vi "stimulate_and_record_async_time.vi"(3 "SSH password":string, 4 "Transfer and Run Date Folder After Experiment":bool, 5 "SSH user name":string, 6 "Tags":string, 7 "Frames":i32, 8 "Convert Power to Voltage":bool, 9 "voltages/power":dbl[](array[numeric]), 10 "parameters":string[](array[string]), 11 "parameters headers":string[](array[string])) -> ()   [LabVIEW 2016]
uses:
  <vilib>/vision/driver/IMAQdx.llb/IMAQdx Acquisition Mode.ctl
  <vilib>/userdefined/High Color/IMAQdx.ctl
  <vilib>/vision/driver/IMAQdx.llb/IMAQdx Buffer Number Mode.ctl
  <vilib>/Utility/file.llb/Write To Spreadsheet File (DBL).vi
  <vilib>/Utility/file.llb/Write To Spreadsheet File (string).vi
  <vilib>/Utility/file.llb/Read From Spreadsheet File (string).vi
  <vilib>/vision/driver/NI_Vision_Acquisition_Software.lvlib
panel:
  out "error out 2":errorcluster
  out "Saved Buffer Number":u32
  out "ProcessFrameRate":dbl
  out "# elements in queue":i32
  out "CameraFrameRate":dbl
  out "Camera Buffer Number":u32
  out "Image":T1(plugin-control)
  out "JPEG Quality":dbl
  out "Save Directory":path
  in  "stop":bool
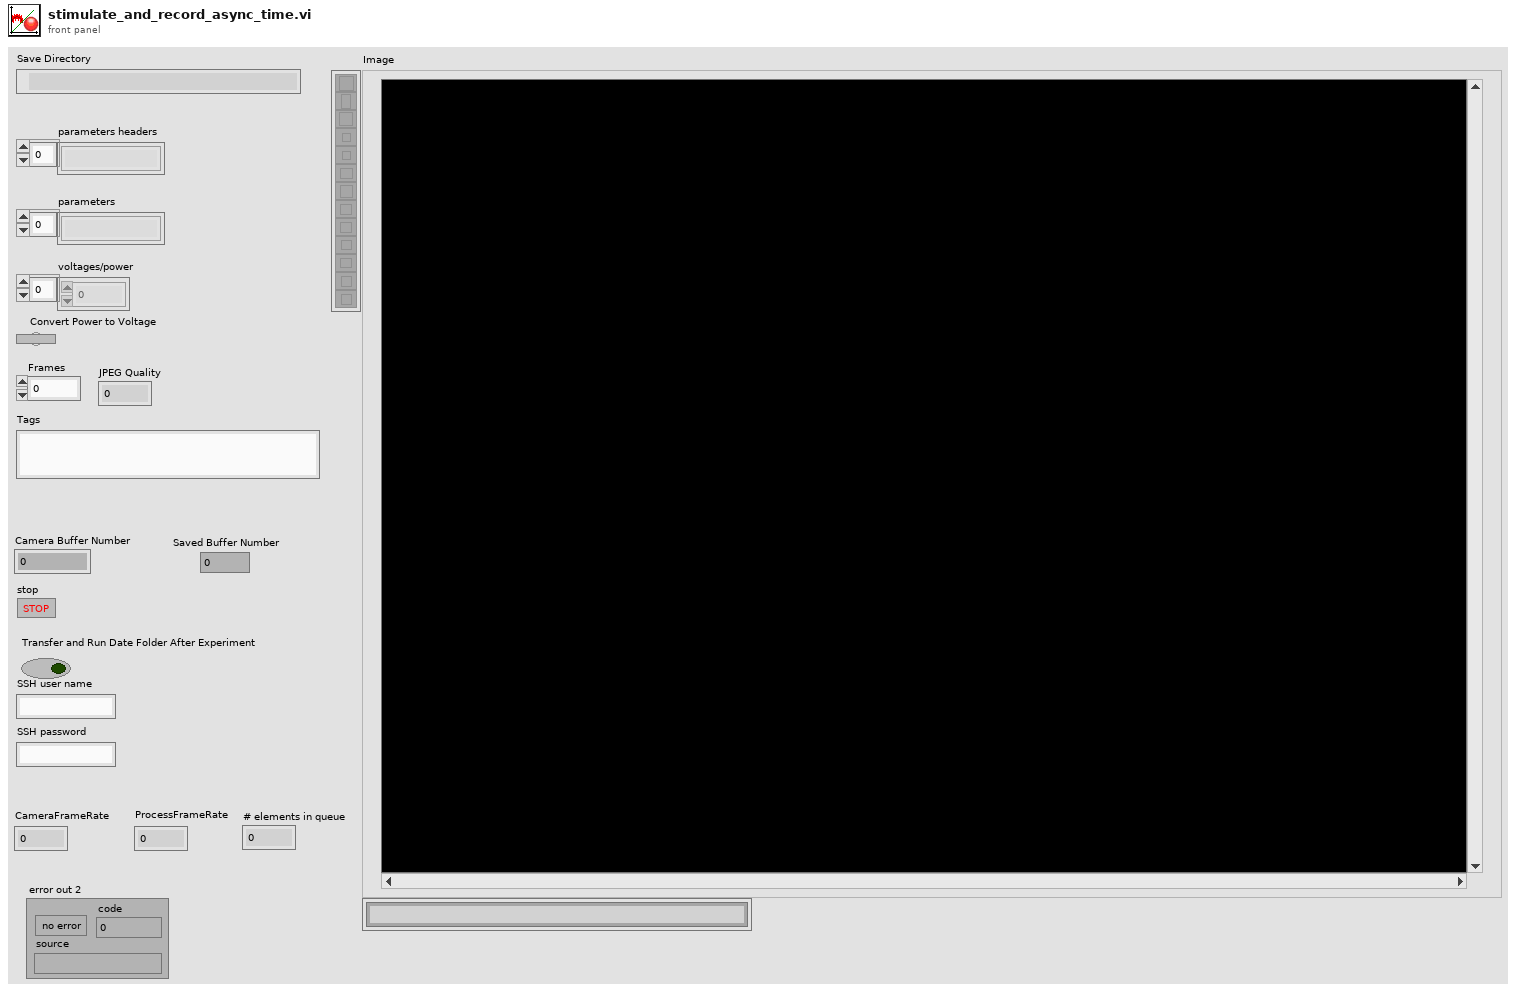
[diagram p1: front panel]
types:
  T1 = typedef "IMAQ Image.ctl" = refnum<image>
  T2 = typedef "IMAQdx.ctl" = refnum<k21>
  T3 = typedef "NI_Vision_Acquisition_Software.lvlib/IMAQdx Buffer Number Mode.ctl" = enum32{"Next", "Last", "Buffer Number", "Every", "Last New"}
  T4 = typedef "Image Type" = u32
  T5 = typedef "NI_Vision_Acquisition_Software.lvlib/IMAQdx Acquisition Mode.ctl" = enum32{"One Shot", "Continuous"}
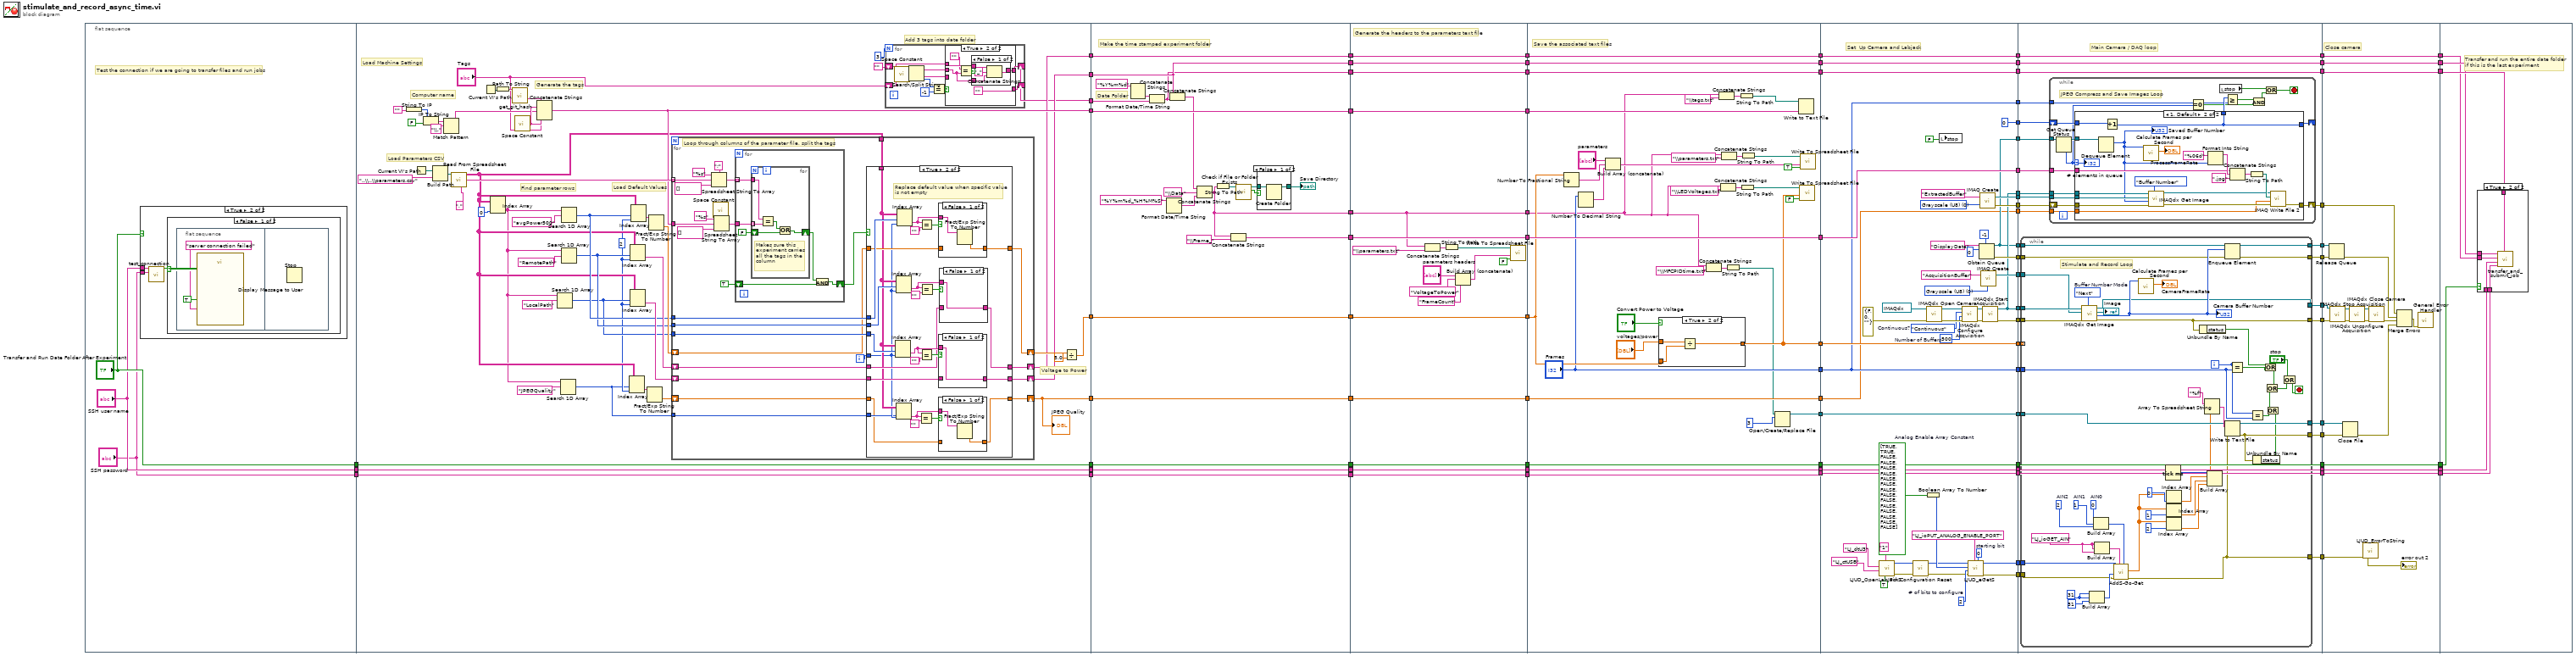
[diagram p0: block diagram]
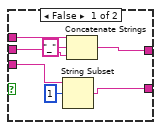
[diagram p4: hidden frame]
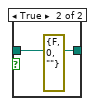
[diagram p11: hidden frame]
diagram:
  n1 = flat-sequence {
    tunnel: ["Transfer and Run Date Folder After Experiment"] -> w54
    tunnel: ["SSH user name"] -> w53
    tunnel: ["SSH password"] -> w52
    tunnel: [w136] -> w84
    tunnel: [w119] -> w83
    tunnel: [w110] -> w74
    tunnel: [w111] -> w73
    tunnel: w54 -> [w128]
    tunnel: w53 -> [w127]
    tunnel: w52 -> [w126]
    tunnel: [w128] -> w45
    tunnel: [w127] -> w38
    tunnel: [w126] -> w37
    tunnel: [w107] -> w30
    tunnel: [w98] -> w29
    tunnel: [w272] -> w68
    tunnel: [w271] -> w66
    tunnel: [w270] -> w64
    tunnel: [w269] -> w62
    tunnel: [w251] -> w60
    tunnel: [w253] -> w58
    tunnel: [w268] -> w56
    tunnel: w73 -> [w268]
    tunnel: w74 -> [w253]
    tunnel: w83 -> [w269]
    tunnel: w84 -> [w270]
    tunnel: [w260] -> w46
    tunnel: w45 -> [w260]
    tunnel: [w259] -> w39
    tunnel: w38 -> [w259]
    tunnel: w37 -> [w258]
    tunnel: [w258] -> w36
    tunnel: w30 -> [w254]
    tunnel: w29 -> [w250]
    tunnel: [w250] -> w26
    tunnel: w68 -> [w294]
    tunnel: [w294] -> w67
    tunnel: w66 -> [w280]
    tunnel: [w280] -> w65
    tunnel: w64 -> [w293]
    tunnel: [w293] -> w63
    tunnel: w62 -> [w292]
    tunnel: [w292] -> w61
    tunnel: w60 -> [w291]
    tunnel: [w291] -> w59
    tunnel: w58 -> [w290]
    tunnel: [w290] -> w57
    tunnel: w56 -> [w289]
    tunnel: [w289] -> w55
    tunnel: [w279] -> w47
    tunnel: w46 -> [w279]
    tunnel: [w278] -> w40
    tunnel: w39 -> [w278]
    tunnel: w36 -> [w277]
    tunnel: [w277] -> w35
    tunnel: [w276] -> w27
    tunnel: w26 -> [w276]
    tunnel: w67 -> [w327]
    tunnel: [w327] -> w89
    tunnel: [w311] -> w87
    tunnel: ["Frames"] -> w86
    tunnel: w65 -> [w295]
    tunnel: w63 -> [w307]
    tunnel: w61 -> [w302]
    tunnel: w59 -> [w316]
    tunnel: [w316] -> w79
    tunnel: [w315] -> w75
    tunnel: w57 -> [w315]
    tunnel: [w314] -> w69
    tunnel: w55 -> [w314]
    tunnel: [w305] -> w48
    tunnel: w47 -> [w305]
    tunnel: [w304] -> w41
    tunnel: w40 -> [w304]
    tunnel: w35 -> [w303]
    tunnel: [w303] -> w34
    tunnel: [w301] -> w28
    tunnel: w27 -> [w301]
    tunnel: [w299] -> w5
    tunnel: w89 -> [w356]
    tunnel: [w383] -> w88
    tunnel: w87 -> [w383]
    tunnel: w86 -> [w355]
    tunnel: [w355] -> w85
    tunnel: [w382] -> w80
    tunnel: w79 -> [w382]
    tunnel: [w381] -> w76
    tunnel: w75 -> [w381]
    tunnel: [w380] -> w70
    tunnel: w69 -> [w380]
    tunnel: [w379] -> w49
    tunnel: w48 -> [w379]
    tunnel: [w378] -> w42
    tunnel: w41 -> [w378]
    tunnel: w34 -> [w377]
    tunnel: [w377] -> w33
    tunnel: w28 -> [w353]
    tunnel: [w349] -> w25
    tunnel: [w357] -> w24
    tunnel: [w361] -> w23
    tunnel: [w360] -> w22
    tunnel: [w354] -> w21
    tunnel: [w359] -> w18
    tunnel: [w358] -> w17
    tunnel: [w357] -> w16
    tunnel: [w356] -> w15
    tunnel: [w355] -> w14
    tunnel: [w354] -> w13
    tunnel: [w353] -> w12
    tunnel: [0] -> w9
    tunnel: w5 -> [w350]
    tunnel: [w350] -> w4
    tunnel: [w339] -> w3
    tunnel: [w334] -> w1
    tunnel: w88 -> [w415]
    tunnel: w85 -> [w414]
    tunnel: [w413] -> w81
    tunnel: w80 -> [w413]
    tunnel: [w412] -> w77
    tunnel: w76 -> [w412]
    tunnel: [w411] -> w71
    tunnel: w70 -> [w411]
    tunnel: [w410] -> w50
    tunnel: w49 -> [w410]
    tunnel: [w409] -> w43
    tunnel: w42 -> [w409]
    tunnel: w33 -> [w408]
    tunnel: [w408] -> w32
    tunnel: w25 -> [w407]
    tunnel: w24 -> [w406]
    tunnel: w23 -> [w405]
    tunnel: w22 -> [w404]
    tunnel: w21 -> [w403]
    tunnel: [w402] -> w20
    tunnel: [w401] -> w19
    tunnel: w18 -> [w400]
    tunnel: w17 -> [w399]
    tunnel: w16 -> [w398]
    tunnel: w15 -> [w397]
    tunnel: w14 -> [w396]
    tunnel: w13 -> [w395]
    tunnel: w12 -> [w394]
    tunnel: [w391] -> w11
    tunnel: [w393] -> w10
    tunnel: w9 -> [w392]
    tunnel: [w390] -> w8
    tunnel: [w389] -> w7
    tunnel: [w388] -> w6
    tunnel: w4 -> [w387]
    tunnel: w3 -> [w386]
    tunnel: [w385] -> w2
    tunnel: w1 -> [w384]
    tunnel: [w526] -> w82
    tunnel: w81 -> [w526]
    tunnel: [w525] -> w78
    tunnel: w77 -> [w525]
    tunnel: [w524] -> w72
    tunnel: w71 -> [w524]
    tunnel: [w523] -> w51
    tunnel: w50 -> [w523]
    tunnel: [w522] -> w44
    tunnel: w43 -> [w522]
    tunnel: w32 -> [w521]
    tunnel: [w521] -> w31
    tunnel: w20 -> [w516]
    tunnel: w19 -> [w515]
    tunnel: w11 -> [w512]
    tunnel: w10 -> [w511]
    tunnel: w8 -> [w510]
    tunnel: w7 -> [w508]
    tunnel: w6 -> [w507]
    tunnel: w2 -> [w506]
    tunnel: w82 -> [w532]
    tunnel: w78 -> [w531]
    tunnel: w72 -> [w530]
    tunnel: w51 -> [w529]
    tunnel: w44 -> [w528]
    tunnel: w31 -> [w527]
    frame #0 {
      # "Test the connection if we are going to transfer files and run jobs"
      n2 = case shown="True" "Transfer and Run Date Folder After Experiment" {
        tunnel: "SSH password" -> [_ w95]
        tunnel: "SSH user name" -> [_ w93]
        frame False {
        }
        frame True {
          n3 = call "test_connection.vi"("Username"=w93, "Password"=w95) -> ("Connection Successful"=w94:bool)  [unwired: 7 in]
          n4 = case shown="False" w94 {
            frame False {
              n5 = flat-sequence {
                frame #0 {
                  n6 = call "Display Message to User"("Enable"=TRUE, "Message"="server connection failed") -> ()  [unwired: 8 in, 2 out]
                }
                frame #1 {
                  n7 = Stop() -> ()  [unwired: 1 in]
                }
              }
            }
            frame True {
            }
          }
        }
      }
    }
    frame #1 {
      w101 = 2
      # "Add 3 tags into date folder"
      # "Generate the tags"
      # "Find parameter rows"
      # "Load Default Values"
      # "Voltage to Power"
      # "Load Parameters CSV"
      # "Computer name"
      # "Load Machine Settings"
      n8 = String To IP(1:"") -> (0:w144:u32)
      n9 = Current VI's Path() -> (path=w139:path)
      n10 = IP To String(1:FALSE, 2:w144) -> (0:w141:string)
      n11 = Build Path(base path=w139, name or relative path="..\\..\\parameters.csv") -> (appended path=w130:path)
      n12 = Match Pattern(string=w141, regular expression="\\.") -> (before substring=w121:string)  [unwired: 1 in, 3 out]
      n13 = call-poly <vilib>:"Read From Spreadsheet File.vi"("delimiter (\\t)"=",", "file path (dialog if empty)"=w130) -> ("first row"=w120:string[], "all rows"=w103:string[][])  [unwired: 5 in, 3 out]
      n14 = Current VI's Path() -> (path=w123:path)
      n15 = Index Array(array=w103, index (col)=0) -> (element=w102:string[])  [unwired: 1 in]
      n16 = Path To String(path=w123) -> (string=w122:string)
      n17 = call "get_git_hash.vi"("VI folder"=w122) -> ("github hash"=w125:string)  [unwired: 10 in]
      n18 = call <vilib>:"Space Constant.vi"() -> ("String"=w124:string)
      n19 = Concatenate Strings(w125, w124, w121, w124, "Tags") -> (w119:string)
      n20 = Search 1D Array(1D array=w102, element="LocalPath") -> (index of element=w113:i32)  [unwired: 1 in]
      n21 = Search 1D Array(1D array=w102, element="JPEGQuality") -> (index of element=w99:i32)  [unwired: 1 in]
      n22 = Search 1D Array(1D array=w102, element="RemotePath") -> (index of element=w114:i32)  [unwired: 1 in]
      n23 = Search 1D Array(1D array=w102, element="avgPower500") -> (index of element=w115:i32)  [unwired: 1 in]
      n24 = Index Array(array=w103, index (row)=w99, index (col)=w101) -> (element=w104:string)
      n25 = Index Array(array=w103, index (row)=w114, index (col)=w101) -> (element=w117:string)
      n26 = Index Array(array=w103, index (row)=w113, index (col)=w101) -> (element=w116:string)
      n27 = Index Array(array=w103, index (row)=w115, index (col)=w101) -> (element=w132:string)
      n28 = Fract/Exp String To Number(string=w104) -> (number=w100:dbl)  [unwired: 3 in, 1 out]
      n29 = Fract/Exp String To Number(string=w132) -> (number=w118:dbl)  [unwired: 3 in, 1 out]
      n30 = for {
        tunnel: w120 -> [w198] mode=indexing
        tunnel: w119 -> [w190]
        tunnel: w115 -> [w185]
        tunnel: w114 -> [w184]
        tunnel: w113 -> [w183]
        tunnel: w103 -> [w188]
        shift-right: [w180] -> w112
        shift-left: w118 -> [w181]
        shift-right: [w177] -> w111
        shift-left: w117 -> [w178]
        shift-right: [w176] -> w110
        shift-left: w116 -> [w179]
        shift-right: [w173] -> w98
        shift-left: w100 -> [w175]
        tunnel: w99 -> [w174]
        i -> [w182]
        # "Loop through columns of the parameter file, split the tags"
        n31 = Spreadsheet String To Array(delimiter (Tab)=";", format string="%s", spreadsheet string=w198, array type (2D Dbl)=string[] []) -> (array=w194:string[])
        n32 = call <vilib>:"Space Constant.vi"() -> ("String"=w192:string)
        n33 = Spreadsheet String To Array(delimiter (Tab)=w192, format string="%s", spreadsheet string=w190, array type (2D Dbl)=string[] []) -> (array=w189:string[])
        n34 = for {
          tunnel: w194 -> [w244] mode=indexing
          tunnel: w189 -> [w243]
          shift-right: [w241] -> w186
          shift-left: TRUE -> [w239]
          n35 = for {
            tunnel: w244 -> [w249]
            tunnel: w243 -> [w248] mode=indexing
            shift-right: [w245] -> w240
            shift-left: FALSE -> [w246]
            # "Makes sure this\nexperiment carries\nall the tags in the\ncolumn"
            n36 = Equal?(x=w249, y=w248) -> (x = y?=w247:bool)
            n37 = Or(x=w247, y=w246) -> (x .or. y?=w245:bool)
          }
          n38 = And(x=w240, y=w239) -> (x .and. y?=w241:bool)
        }
        n39 = case shown="True" w186 {
          tunnel: w181 -> [w202 w223]
          tunnel: [w202 w222] -> w180
          tunnel: w185 -> [_ w228]
          tunnel: w184 -> [_ w227]
          tunnel: w183 -> [_ w226]
          tunnel: w182 -> [_ w205]
          tunnel: w188 -> [_ w206]
          tunnel: [w201 w212] -> w177
          tunnel: [w200 w214] -> w176
          tunnel: w179 -> [w200 w213]
          tunnel: w178 -> [w201 w211]
          tunnel: w175 -> [w199 w203]
          tunnel: w174 -> [_ w204]
          tunnel: [w199 w207] -> w173
          frame False {
          }
          frame True {
            # "Replace default value when specific value\nis not empty"
            n40 = Index Array(array=w206, index (row)=w226, index (col)=w205) -> (element=w215:string)
            n41 = Index Array(array=w206, index (row)=w227, index (col)=w205) -> (element=w218:string)
            n42 = Index Array(array=w206, index (row)=w204, index (col)=w205) -> (element=w208:string)
            n43 = Index Array(array=w206, index (row)=w228, index (col)=w205) -> (element=w221:string)
            n44 = Equal?(x=w208, y="") -> (x = y?=w209:bool)
            n45 = Equal?(x=w221, y="") -> (x = y?=w224:bool)
            n46 = Equal?(x=w215, y="") -> (x = y?=w216:bool)
            n47 = Equal?(x=w218, y="") -> (x = y?=w219:bool)
            n48 = case shown="False" w209 {
              tunnel: w203 -> [_ w231]
              tunnel: [w230 w231] -> w207
              tunnel: w208 -> [w229 _]
              frame False {
                n49 = Fract/Exp String To Number(string=w229) -> (number=w230:dbl)  [unwired: 3 in, 1 out]
              }
              frame True {
              }
            }
            n50 = case shown="False" w224 {
              tunnel: w223 -> [_ w238]
              tunnel: [w237 w238] -> w222
              tunnel: w221 -> [w236 _]
              frame False {
                n51 = Fract/Exp String To Number(string=w236) -> (number=w237:dbl)  [unwired: 3 in, 1 out]
              }
              frame True {
              }
            }
            n52 = case shown="False" w216 {
              tunnel: w215 -> [w232 _]
              tunnel: [w232 w233] -> w214
              tunnel: w213 -> [_ w233]
              frame False {
              }
              frame True {
              }
            }
            n53 = case shown="False" w219 {
              tunnel: w218 -> [w234 _]
              tunnel: [w234 w235] -> w212
              tunnel: w211 -> [_ w235]
              frame False {
              }
              frame True {
              }
            }
          }
        }
      }
      "JPEG Quality" <- w98
      n54 = for {
        N: 3 -> [_]
        shift-right: [w145] -> _
        shift-left: "Tags" -> [w154]
        shift-right: [w147] -> w107
        shift-left: "" -> [w152]
        n55 = call <vilib>:"Space Constant.vi"() -> ("String"=w153:string)
        n56 = Search/Split String(string=w154, search string/char (-)=w153) -> (substring before match=w151:string, match + rest of string=w150:string, offset of match=w149:i32)  [unwired: 1 in]
        n57 = Equal?(x=w149, y=-1) -> (x = y?=w146:bool)
        n58 = case shown="True" w146 {
          tunnel: w152 -> [w155 w165]
          tunnel: w151 -> [w156 w162]
          tunnel: w150 -> [w157 _]
          tunnel: [w159 ""] -> w145
          tunnel: [w158 w164] -> w147
          frame False {
            n59 = String Subset(string=w157, offset (0)=1) -> (substring=w159:string)  [unwired: 1 in]
            n60 = Concatenate Strings(w155, "_", w156) -> (w158:string)
          }
          frame True {
            n61 = Equal?(x="", y=w162) -> (x = y?=w166:bool)
            n62 = case shown="False" w166 {
              tunnel: w165 -> [w169 w172]
              tunnel: [w170 w172] -> w164
              tunnel: w162 -> [w168 _]
              frame False {
                n63 = Concatenate Strings(w169, "_", w168) -> (w170:string)
              }
              frame True {
              }
            }
          }
        }
      }
      n64 = Divide(x=w112, y=5.0) -> (x/y=w136:dbl)
    }
    frame #2 {
      # "Make the time stamped experiment folder"
      # "Date Folder"
      n65 = Format Date/Time String(time format string (%c)="%Y%m%d") -> (date/time string=w255:string)  [unwired: 2 in]
      n66 = Concatenate Strings(w255, w254) -> (w251:string)
      n67 = Format Date/Time String(time format string (%c)="%Y%m%d_%H%M%S") -> (date/time string=w257:string)  [unwired: 2 in]
      n68 = Concatenate Strings(w253, w251) -> (w252:string)
      n69 = Concatenate Strings(w252, "\\Data", w257) -> (w271:string)
      n70 = String To Path(string=w271) -> (path=w263:path)
      n71 = Concatenate Strings(w271, "\\Frame_") -> (w272:string)
      n72 = call <vilib>:"Check if File or Folder Exists.vi"("path"=w263) -> ("file or folder exists?"=w266:bool, "dup path"=w265:path)  [unwired: 8 in, 1 out]
      n73 = case shown="False" w266 {
        tunnel: [w273 w275] -> w262
        tunnel: w265 -> [w274 w275]
        frame False {
          n74 = Create Folder(path (use dialog)=w274) -> (created path=w273:path)  [unwired: 2 in, 2 out]
        }
        frame True {
          (unwired) errorcluster {"status"=FALSE, "code"=0, "source"=""} ("error out")
        }
      }
      "Save Directory" <- w262
    }
    frame #3 {
      # "Generate the headers to the parameters text file"
      n75 = Concatenate Strings(w280, "\\parameters.txt") -> (w288:string)
      n76 = String To Path(string=w288) -> (path=w287:path)
      n77 = Build Array (concatenate)("parameters headers", "VoltageToPower", "FrameCount") -> (w284:string[])
      n78 = call-poly <vilib>:"Write To Spreadsheet File.vi"("append to file? (new file:F)"=FALSE, "1D data"=w284, "file path (dialog if empty)"=w287) -> ()  [unwired: 5 in, 1 out]
    }
    frame #4 {
      # "Save the associated text files"
      n79 = Number To Fractional String(number=w307) -> (F-format string=w308:string)  [unwired: 3 in]
      n80 = Number To Decimal String(number="Frames") -> (decimal integer string=w309:string)  [unwired: 1 in]
      n81 = Build Array (concatenate)("parameters", w308, w309) -> (w320:string[])
      n82 = case shown="True" "Convert Power to Voltage" {
        tunnel: "voltages/power" -> [w330 w333]
        tunnel: [w330 w331] -> w311
        tunnel: w307 -> [_ w332]
        frame False {
        }
        frame True {
          n83 = Divide(x=w333, y=w332) -> (x/y=w331:dbl[])
        }
      }
      n84 = Concatenate Strings(w295, "\\MFCPIDtime.txt") -> (w298:string)
      n85 = Concatenate Strings(w295, "\\tags.txt") -> (w318:string)
      n86 = Concatenate Strings(w295, "\\LEDVoltages.txt") -> (w329:string)
      n87 = Concatenate Strings(w295, "\\parameters.txt") -> (w324:string)
      n88 = String To Path(string=w298) -> (path=w296:path)
      n89 = String To Path(string=w318) -> (path=w317:path)
      n90 = String To Path(string=w329) -> (path=w328:path)
      n91 = String To Path(string=w324) -> (path=w323:path)
      n92 = Open/Create/Replace File(file path (use dialog)=w296, operation (0:open)=3) -> (refnum out=w299:refnum<file>)  [unwired: 4 in, 2 out]
      n93 = Write to Text File(file (use dialog)=w317, text=w302) -> ()  [unwired: 2 in, 3 out]
      n94 = call-poly <vilib>:"Write To Spreadsheet File.vi"("append to file? (new file:F)"=FALSE, "1D data"=w311, "file path (dialog if empty)"=w328) -> ()  [unwired: 5 in, 1 out]
      n95 = call-poly <vilib>:"Write To Spreadsheet File.vi"("append to file? (new file:F)"=TRUE, "1D data"=w320, "file path (dialog if empty)"=w323) -> ()  [unwired: 5 in, 1 out]
    }
    frame #5 {
      w347 = 2  # # of bits to configure
      w345 = 0  # starting bit
      w344 = bool[] [TRUE, TRUE, FALSE, FALSE, FALSE, FALSE, FALSE, FALSE, FALSE, FALSE, FALSE, FALSE, FALSE, FALSE, FALSE, FALSE]  # Analog Enable Array Constant
      w364 = T4 0 items=["Grayscale (U8)", "Grayscale (I16)", "Grayscale (SGL)", "Complex (CSG)", "RGB (U32)", "HSL (U32)", "RGB (U64)"] ("Image Type")
      w373 = T4 0 items=["Grayscale (U8)", "Grayscale (I16)", "Grayscale (SGL)", "Complex (CSG)", "RGB (U32)", "HSL (U32)", "RGB (U64)"] ("Image Type")
      w374 = u32 500  # Number of Buffers
      w370 = IMAQdx_Acquisition_Mode."Continuous"  # Continuous?
      # "Set  Up Camera and Labjack"
      n96 = call "LJUD_OpenLabJackS.vi"("FirstFound"=TRUE, "Address"="1", "ConnectionType"="LJ_ctUSB", "DeviceType"="LJ_dtU3") -> ("error out"=w336:errorcluster, "Handle"=w338:i32)  [unwired: 5 in, 1 out]
      n97 = call "Pin Configuration Reset.vi"("error in"=w336, "Handle In"=w338) -> ("error out"=w335:errorcluster, "Handle Out"=w337:i32)  [unwired: 8 in]
      n98 = Boolean Array To Number(Boolean array=w344) -> (number=w348:u32)
      n99 = call <vilib>:"IMAQdx Open Camera.vi"("error in"=errorcluster {"status"=FALSE, "code"=0, "source"=""}, "Session In"=T2 "cam0") -> ("error out"=w375:errorcluster, "Session Out"=w376:T2)  [unwired: 8 in]
      n100 = local write "stop"(FALSE) -> ()
      n101 = call <vilib>:"IMAQdx Configure Acquisition.vi"("error in"=w375, "Number of Buffers"=w374, "Continuous?"=w370, "Session In"=w376) -> ("error out"=w371:errorcluster, "Session Out"=w369:T2)  [unwired: 6 in]
      n102 = call "LJUD_eGetS.vi"("Channel"=w345, "IOType"="LJ_ioPUT_ANALOG_ENABLE_PORT", "error in"=w335, "x1"=w347, "Value Write"=w348, "Handle In"=w337) -> ("error out"=w339:errorcluster, "Handle Out"=w334:i32)  [unwired: 3 in, 1 out]
      n103 = Obtain Queue(max queue size (-1, unlimited)=-1, name (unnamed)="DisplayData", element data type=u32 0) -> (queue out=w354:refnum<queue>, error out=w360:errorcluster)  [unwired: 2 in, 1 out]
      n104 = call "IMAQ Create"("Image Name"="ExtractedBuffer", "Image Type"=w364) -> ("New Image"=w358:T1, "error out"=w359:errorcluster)  [unwired: 3 in]
      n105 = call "IMAQ Create"("Image Name"="AcquisitionBuffer", "Image Type"=w373) -> ("New Image"=w361:T1)  [unwired: 3 in, 1 out]
      n106 = call <vilib>:"IMAQdx Start Acquisition.vi"("error in"=w371, "Session In"=w369) -> ("error out"=w349:errorcluster, "Session Out"=w357:T2)  [unwired: 8 in]
    }
    frame #6 {
      # "Main Camera / DAQ loop"
      n107 = while {
        tunnel: w415 -> [_] mode=indexing
        tunnel: w414 -> [w460]
        tunnel: w407 -> [w501]
        tunnel: w406 -> [w500]
        tunnel: w405 -> [w499]
        tunnel: w404 -> [w498]
        tunnel: w403 -> [w497]
        tunnel: [w494] -> w390
        tunnel: [w493] -> w391
        tunnel: [w492] -> w402
        tunnel: [w491] -> w401
        tunnel: [w465] -> w389
        tunnel: [w487] -> w388
        tunnel: w387 -> [w486]
        tunnel: w386 -> [w467]
        tunnel: [w466] -> w385
        tunnel: w384 -> [w456]
        i -> [w461]
        stop <- w459 stop-if-true
        w477 = 2  # AIN2
        w473 = 31 ("AIN0")
        w481 = 1  # AIN1
        w480 = 0  # AIN0
        w474 = "LJ_ioGET_AIN" ("IOType")
        w505 = IMAQdx_Buffer_Number_Mode."Next"  # Buffer Number Mode
        # "Stimulate and Record Loop"
        n108 = call <vilib>:"IMAQdx Get Image.vi"("Buffer Number Mode (Next)"=w505, "error in"=w501, "Image In"=w499, "Session In"=w500) -> ("error out"=w491:errorcluster, "Buffer Number Out"=w502:u32, "Image Out"=→"Image":T1, "Session Out"=w492:T2)  [unwired: 4 in]
        "Camera Buffer Number" <- w502
        n109 = Build Array(w473, w473, 31 ("AIN1")) -> (w478:i32[])
        n110 = Build Array(w480, w481, w477) -> (w484:i32[])
        n111 = Build Array(w474, w474, w474) -> (w485:string[])
        n112 = call "AddS-Go-Get.vi"("Channels"=w484, "IOTypes"=w485, "error in"=w467, "x1"=w478, "Handle In"=w456) -> ("error out"=w466:errorcluster, "Values Read"=w475:dbl[])  [unwired: 4 in, 1 out]
        n113 = call <vilib>:"Calculate Frames per Second.vi"("Buffer Number"=w502) -> ("Processed Frames/s"=→"CameraFrameRate":dbl)  [unwired: 8 in, 2 out]
        n114 = Tick Count (ms)() -> (millisecond timer value=w472:u32)
        n115 = Index Array(array=w475, index=0 ("Index")) -> (element=w470:dbl)
        n116 = Index Array(array=w475, index=1 ("Index")) -> (element=w469:dbl)
        n117 = Index Array(array=w475, index=2 ("Index")) -> (element=w468:dbl)
        n118 = Unbundle By Name(w491) -> ("status"=w496:bool)
        n119 = Build Array(w472, w470, w469, w468) -> (w471:dbl[])
        n120 = Array To Spreadsheet String(array=w471, 3:"%f") -> (spreadsheet string=w489:string)  [unwired: 1 in]
        n121 = Enqueue Element(queue=w497, element=w502, error in (no error)=w498) -> (queue out=w494:refnum<queue>, error out=w493:errorcluster)  [unwired: 1 in, 1 out]
        n122 = Write to Text File(file (use dialog)=w486, text=w489, error in=w466) -> (refnum out=w487:refnum<file>, error out=w465:errorcluster)  [unwired: 1 in, 1 out]
        n123 = Equal?(x=w461, y=w460) -> (x = y?=w490:bool)
        n124 = Equal?(x=w461, y=w460) -> (x = y?=w462:bool)
        n125 = Unbundle By Name(w465) -> ("status"=w464:bool)
        n126 = Or(x=w496, y=w490) -> (x .or. y?=w495:bool)
        n127 = Or(x=w462, y=w464) -> (x .or. y?=w463:bool)
        n128 = Or(x=w495, y=w463) -> (x .or. y?=w457:bool)
        n129 = Or(x="stop", y=w457) -> (x .or. y?=w459:bool)
      }
      n130 = while {
        tunnel: w395 -> [w433]
        tunnel: w399 -> [w431]
        tunnel: w398 -> [w430]
        tunnel: w397 -> [w428]
        shift-right: [w427] -> w393
        shift-left: w400 -> [w429]
        tunnel: w396 -> [w420]
        tunnel: w394 -> [w425]
        shift-right: [w422] -> _
        shift-left: w392 -> [w423]
        stop <- w426 stop-if-true
        # "JPEG Compress and Save Images Loop"
        n131 = Get Queue Status(queue=w433) -> (queue out=w432:refnum<queue>, # elements in queue=w416:i32)  [unwired: 2 in, 6 out]
        n132 = case shown="1, Default" w416 {
          selector: w416 -> [_ w454]
          tunnel: w432 -> [_ w452]
          tunnel: w431 -> [_ w451]
          tunnel: w430 -> [_ w450]
          tunnel: w429 -> [w435 w449]
          tunnel: w428 -> [_ w443]
          tunnel: [w435 w439] -> w427
          tunnel: w425 -> [_ w438]
          tunnel: w423 -> [w434 w437]
          tunnel: [w434 w436] -> w422
          tunnel: [w434 w436] -> w421
          frame 0 {
          }
          frame 1, Default {
            n133 = Dequeue Element(queue=w452) -> (element=w440:u32)  [unwired: 2 in, 3 out]
            "Saved Buffer Number" <- w440
            n134 = Increment(x=w437) -> (x+1=w436:i32)
            n135 = call <vilib>:"Calculate Frames per Second.vi"("Buffer Number"=w440) -> ("Processed Frames/s"=→"ProcessFrameRate":dbl)  [unwired: 8 in, 2 out]
            n136 = call <vilib>:"IMAQdx Get Image.vi"("Buffer Number Mode (Next)"=IMAQdx_Buffer_Number_Mode."Buffer Number", "error in"=w449, "Buffer Number In"=w440, "Image In"=w451, "Session In"=w450) -> ("error out"=w441:errorcluster, "Image Out"=w442:T1)  [unwired: 3 in, 2 out]
            n137 = Format Into String(format string="%06d" ("string"), w440) -> (resulting string=w445:string)  [unwired: 2 in, 1 out]
            n138 = Concatenate Strings(w443, w445, ".jpg" ("string")) -> (w447:string)
            n139 = String To Path(string=w447) -> (path=w446:path)
            n140 = call-poly "IMAQ Write File 2"("error in (no error)"=w441, "Image Quality"=w438, "File Path"=w446, "Image"=w442) -> ("error out"=w439:errorcluster)  [unwired: 6 in, 1 out]
            "# elements in queue" <- w454
          }
        }
        n141 = Equal To 0?(x=w416) -> (x = 0?=w417:bool)
        n142 = local read "stop"() -> (w424:bool)
        n143 = Greater Or Equal?(x=w421, y=w420) -> (x >= y?=w419:bool)
        n144 = And(x=w419, y=w417) -> (x .and. y?=w418:bool)
        n145 = Or(x=w424, y=w418) -> (x .or. y?=w426:bool)
      }
    }
    frame #7 {
      # "Close camera"
      n146 = Release Queue(queue=w510) -> ()  [unwired: 2 in, 3 out]
      n147 = call <vilib>:"IMAQdx Stop Acquisition.vi"("error in"=w515, "Session In"=w516) -> ("error out"=w517:errorcluster, "Session Out"=w518:T2)  [unwired: 8 in]
      n148 = Close File(refnum=w507, error in=w508) -> (error out=w509:errorcluster)  [unwired: 1 out]
      n149 = call <vilib>:"IMAQdx Unconfigure Acquisition.vi"("error in"=w517, "Session In"=w518) -> ("error out"=w520:errorcluster, "Session Out"=w519:T2)  [unwired: 8 in]
      n150 = call "LJUD_ErrorToString.vi"("error in"=w506) -> ()  [unwired: 10 in, 1 out]
      n151 = call <vilib>:"IMAQdx Close Camera.vi"("error in"=w520, "Session In"=w519) -> ("error out"=w513:errorcluster)  [unwired: 9 in]
      n152 = Merge Errors(w511, w512, w513, w509) -> (w514:errorcluster)
      n153 = call <vilib>:"General Error Handler.vi"("error in (no error)"=w514) -> ()  [unwired: 10 in, 5 out]
      "error out 2" <- w506
    }
    frame #8 {
      # "Transfer and run the entire date folder\nif this is the last experiment"
      n154 = case shown="True" w529 {
        tunnel: w532 -> [_ w537]
        tunnel: w531 -> [_ w536]
        tunnel: w530 -> [_ w535]
        tunnel: w528 -> [_ w534]
        tunnel: w527 -> [_ w533]
        frame False {
        }
        frame True {
          n155 = call "transfer_and_submit_job.vi"("Date Folder"=w537, "Password"=w533, "Username"=w534, "Remote Data Directory"=w535, "Local Data Directory"=w536) -> ()  [unwired: 7 in]
        }
      }
    }
  }
